vi "Example Array 1.vi"(8 "Error In":errorcluster) -> (0 "Error Out":errorcluster, 3 "current array element":i32)   [LabVIEW 2018]
panel:
  out "array w/ subset deleted":dbl[](array[numeric])
  out "size(s)":i32
  out "output array":dbl[](array[numeric])
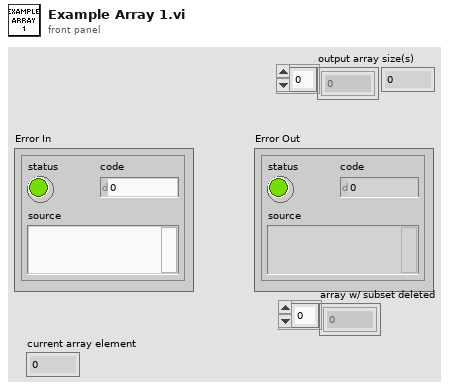
[diagram p1: front panel]
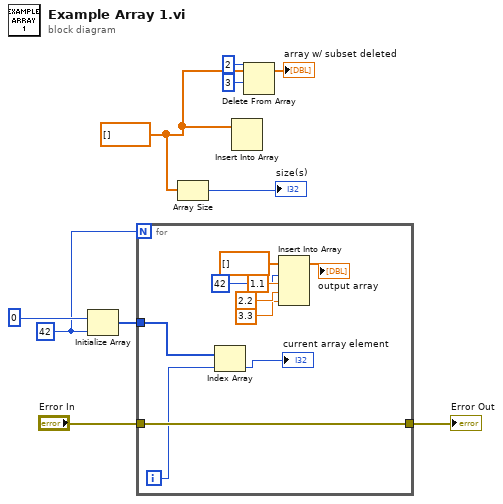
[diagram p0: block diagram]
diagram:
  w4 = dbl[] [] ("array")
  w6 = 42 ("dimension size")
  n1 = Initialize Array "Initialize Array"(0, w6) -> (w9:i32[])
  n2 = for {
    N: w6 -> [_]
    tunnel: w9 -> [w19]
    tunnel: [w20] -> w8
    tunnel: "Error In" -> [w20]
    i -> [w18]
    n3 = Index Array "Index Array"(array=w19, index=w18) -> (element=→"current array element":i32)
    n4 = Insert Into Array(array=dbl[] [], index=42, new element #1=1.1 ("new element/subarray"), new element #2=2.2 ("new element/subarray"), new element #3=3.3 ("new element/subarray")) -> (→"output array":dbl[])
  }
  "Error Out" <- w8
  n5 = Array Size(array=w4) -> (size(s)=→"size(s)":i32)
  n6 = Insert Into Array(array=w4) -> ()  [unwired: 2 in, 1 out]
  n7 = Delete From Array(array=w4, length=3, index=2) -> (array with subset deleted=→"array w/ subset deleted":dbl[])  [unwired: 1 out]
